vi "Create DAQmx.vi"(8 "error in (no error)":errorcluster, 10 "Configuration":T1={"Channels"="", "DAQType"=enum."AI", "minimum value"=-5.0, "maximum value"=5.0, "sampling info"={"Fs"=0.0, "#s"=0.0}, "SamplingMode"=enum."Continuous"} {"maximum value" format="%0.2f"; "minimum value" format="%0.2f"}, 11 "DAQmx in":refnum<class "DAQmx.lvclass">) -> (0 "error out":errorcluster, 3 "DAQmx out":refnum<class "DAQmx.lvclass">)   [LabVIEW 2016, in "DAQmx.lvclass"]
uses:
  DAQmx.lvclass
  C:/user/patrick/hg/lockin.SMO/lvsrc/DAQ/DAQ.lvclass
  DAQ/Typedefs/DAQ.Config.ctl
  DAQ/Typedefs/PrivateEvents--DAQ.AI.Channels.ctl
  DAQ/Typedefs/DAQType.ctl
  DAQ/Typedefs/SamplingInfo.ctl
  DAQ/Typedefs/SamplingMode.ctl
  DAQ/DAQ.lvclass
panel:
  # "Specific DAQmx config\nWire it to the connector pane"
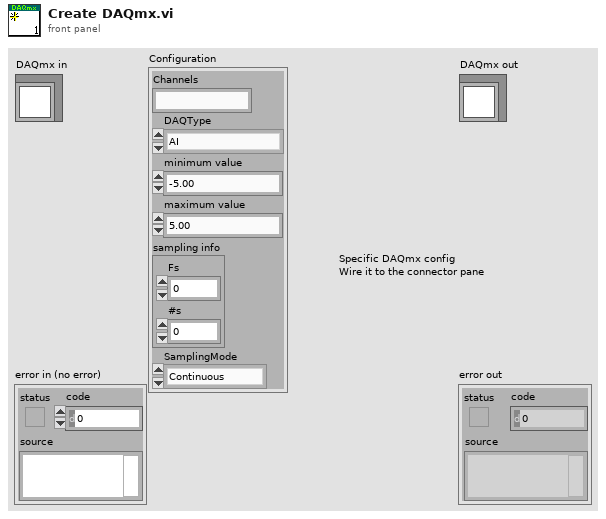
[diagram p1: front panel]
types:
  T1 = typedef "DAQ.lvclass/DAQ.Config.ctl" = cluster{"Channels":T2, "DAQType":T3, "minimum value":dbl, "maximum value":dbl, "sampling info":T4, "SamplingMode":T5}
  T2 = typedef "PrivateEvents--DAQ.AI.Channels.ctl" = string
  T3 = typedef "DAQ.lvclass/DAQType.ctl" = enum16{"AI", "AO"}
  T4 = typedef "DAQ.lvclass/SamplingInfo.ctl" = cluster{"Fs":dbl, "#s":dbl}
  T5 = typedef "DAQ.lvclass/SamplingMode.ctl" = enum16{"Continuous", "Finite"}
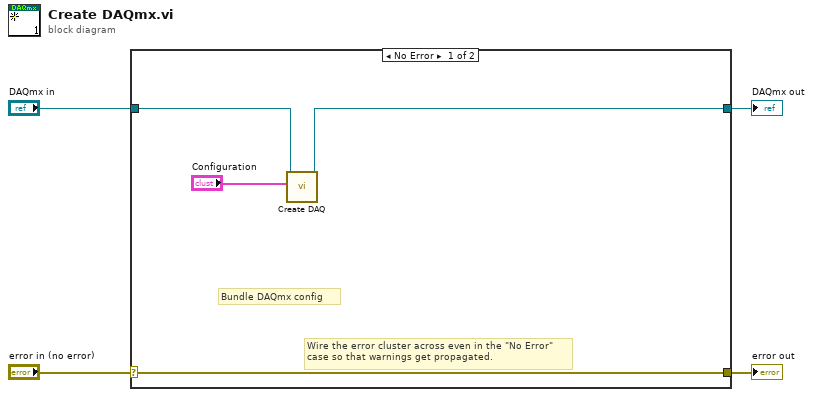
[diagram p0: block diagram]
diagram:
  n1 = case shown="No Error" "error in (no error)" {
    selector: "error in (no error)" -> [w8 w10]
    tunnel: [w8 w10] -> w3
    tunnel: [w5 w9] -> w1
    tunnel: "DAQmx in" -> [w7 w9]
    frame No Error {
      # "Bundle DAQmx config"
      # "Wire the error cluster across even in the \"No Error\"\ncase so that warnings get propagated."
      n2 = call "Create DAQ.vi"("Configuration"="Configuration", "DAQ in"=w7) -> ("DAQ out"=w5:refnum<class "DAQmx.lvclass">)  [unwired: 8 in, 1 out]
    }
    frame Error {
    }
  }
  "error out" <- w3
  "DAQmx out" <- w1
